vi "HandShaking.vi"(6 "Elapsed Time":u32, 8 "error in":errorcluster, 10 "Event Sources":T1, 11 "Ignition in":refnum<class "Ignition.lvclass">) -> (0 "error out":errorcluster, 3 "Ignition out":refnum<class "Ignition.lvclass">)   [LabVIEW 2021, in "Ignition.lvclass"]
uses:
  Ignition.lvclass
  Ignition.lvclass/Ignition.ctl
  <vilib>/addons/TestStand/_TSUtility.llb/TestStand - Get Property Value (String).vi
  OPC UA/OPC UA.lvclass
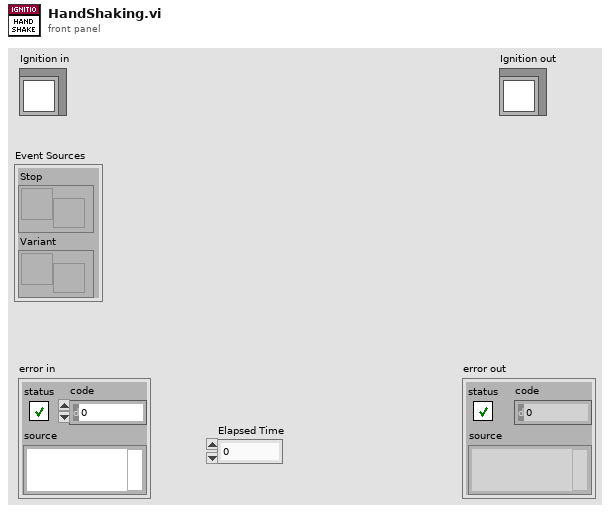
[diagram p1: front panel]
types:
  T1 = cluster{"Stop":refnum<user-event>, "Variant":refnum<user-event>}
  T2 = typedef "Ignition.lvclass/Tester Rx.ctl" = cluster{"result_ack":bool}
  T3 = typedef "Ignition.lvclass/Tester Tx.ctl" = cluster{"thermistor":dbl, "phase_angle":dbl, "pallet_rfid":dbl, "ocv":dbl, "cell_vsense1":dbl, "cell_vsense2":dbl, "hipot1_leakage_current":dbl, "hipot2_leakage_current":dbl, "guid":string, "can_sn":string, "can_pn":string, "ac_internal_resistance":dbl, "sub_station":string, "fault_code":i32, "elapsed_time":i32, "result":i32, "reject_code_reason":string, "result_ready":bool, "Timeout":bool}
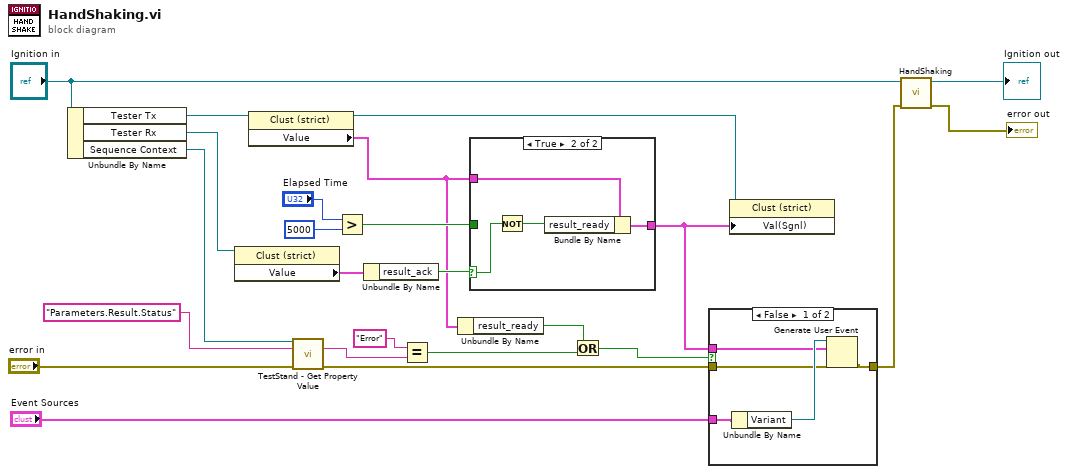
[diagram p0: block diagram]
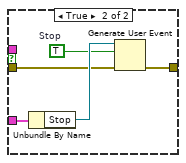
[diagram p2: hidden frame]
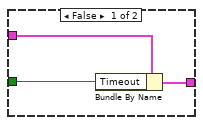
[diagram p3: hidden frame]
diagram:
  n1 = Unbundle By Name("Ignition in") -> ("Tester Tx"=w21:refnum<vi>, "Tester Rx"=w16:refnum<vi>, "Sequence Context"=w9:refnum<k7>)
  n2 = property class="Clust (strict)"(reference=w16) -> ("Value"=w15:T2)  [unwired: 1 in, 2 out]
  n3 = property class="Clust (strict)"(reference=w21) -> (reference out=w20:refnum<vi>, "Value"=w2:T3)  [unwired: 1 in, 1 out]
  n4 = call-poly <vilib>:"TestStand - Get Property Value.vi"("Sequence Context In"=w9, "Lookup String"="Parameters.Result.Status", "error in (no error)"="error in") -> ("Value"=w10:string, "error out"=w6:errorcluster)  [unwired: 10 in, 1 out]
  n5 = Greater?(x="Elapsed Time", y=u32 5000) -> (0:w17:bool)
  n6 = Unbundle By Name(w15) -> ("result_ack"=w3:bool)
  n7 = Equal?(x="Error" ("Lookup String"), y=w10) -> (x = y?=w5:bool)
  n8 = Unbundle By Name(w2) -> ("result_ready"=w1:bool)
  n9 = case shown="True" w3 {
    selector: w3 -> [_ w29]
    tunnel: w2 -> [w27 w31]
    tunnel: [w26 w30] -> w14
    tunnel: w17 -> [w25 _]
    frame False {
      n10 = Bundle By Name(cluster=w27, "Timeout"=w25) -> (w26:T3)
    }
    frame True {
      n11 = Not(x=w29) -> (.not. x?=w28:bool)
      n12 = Bundle By Name(cluster=w31, "result_ready"=w28) -> (w30:T3)
    }
  }
  n13 = Or(x=w1, y=w5) -> (x .or. y?=w4:bool)
  n14 = case shown="False" w4 {
    tunnel: "Event Sources" -> [w36 w41]
    tunnel: w14 -> [w34 _]
    tunnel: w6 -> [w33 w38]
    tunnel: [w32 w37] -> w12
    frame False {
      n15 = Unbundle By Name(w36) -> ("Variant"=w35:refnum<user-event>)
      n16 = Generate User Event(user event=w35, event data cluster=w34, error in=w33) -> (error out=w32:errorcluster)  [unwired: 1 in, 1 out]
    }
    frame True {
      w39 = TRUE  # Stop
      n17 = Unbundle By Name(w41) -> ("Stop"=w40:refnum<user-event>)
      n18 = Generate User Event(user event=w40, event data cluster=w39, error in=w38) -> (error out=w37:errorcluster)  [unwired: 1 in, 1 out]
    }
  }
  n19 = property class="Clust (strict)"(reference=w20, "Val(Sgnl)"=w14) -> ()  [unwired: 1 in, 2 out]
  n20 = call-parent "HandShaking.vi"("error in (no error)"=w12, "OPC UA in"="Ignition in") -> ("error out"=→"error out":errorcluster, "OPC UA out"=→"Ignition out":refnum<class "Ignition.lvclass">)  [unwired: 8 in]
